vi "RT Loop - System Health and FPGA Monitoring.vi"(10 "FPGA VI Reference Out 2":refnum<k20>, 11 "Message Queue":refnum<queue>) -> (3 "x*y":dbl)   [LabVIEW 2017]
doc: "Send RT diagnostic information and FPGA monitoring data to UI Main VI."
uses:
  UI Error Handlers/support/Message Queue/Message Cluster.ctl
  controls/CPU Loads.ctl
  controls/FPGA State.ctl
  Globals/Global - Configuration Options.vi
  Globals/Global - All RT Loop Stop.vi
  <vilib>/Utility/error.llb/Error Cluster From Error Code.vi
  <vilib>/rvi/errors/niLvFpgaAdjustHostInterfaceError.vi
  <vilib>/nisyscfg/Close (System).vi
  <vilib>/rvi/interface/nirviReadWriteControl/nirviReadWriteControl.xnode
  <vilib>/NI_Real-Time Target Support.lvlib
  <vilib>/nisyscfg/nisyscfg.lvlib
  <resource>/objmgr/nisysapi.rc
  NiFpgaLv.dll
  <vilib>/rvi/interface/Simulation/niFpgaSimulationCallBeginRW.vi
  UI Error Handlers/support/Message Queue/Message Queue.lvlib
panel:
  out "x = y?":bool
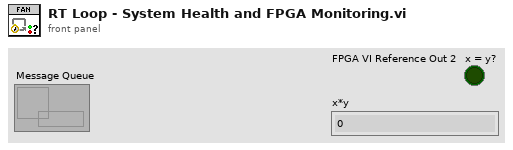
[diagram p1: front panel]
types:
  T1 = typedef "NI_Real-Time Target Support.lvlib/RT CPU Load.ctl" = cluster{"Total (%)":dbl, "Time Critical (%)":dbl, "Timed Structures (%)":dbl, "High (%)":dbl, "Above Normal (%)":dbl, "Normal (%)":dbl, "Background (%)":dbl, "Idle (%)":dbl, "ISR (%)":dbl}
  T2 = cluster{"Tool data":cluster{"Number of teeth":sgl}, "Cutting data":cluster{"rpm":sgl}, "Limits":cluster{"Magnitude threshold":sgl, "Tolerance":sgl}, "G1 status":cluster{"G1 trigger":bool}}
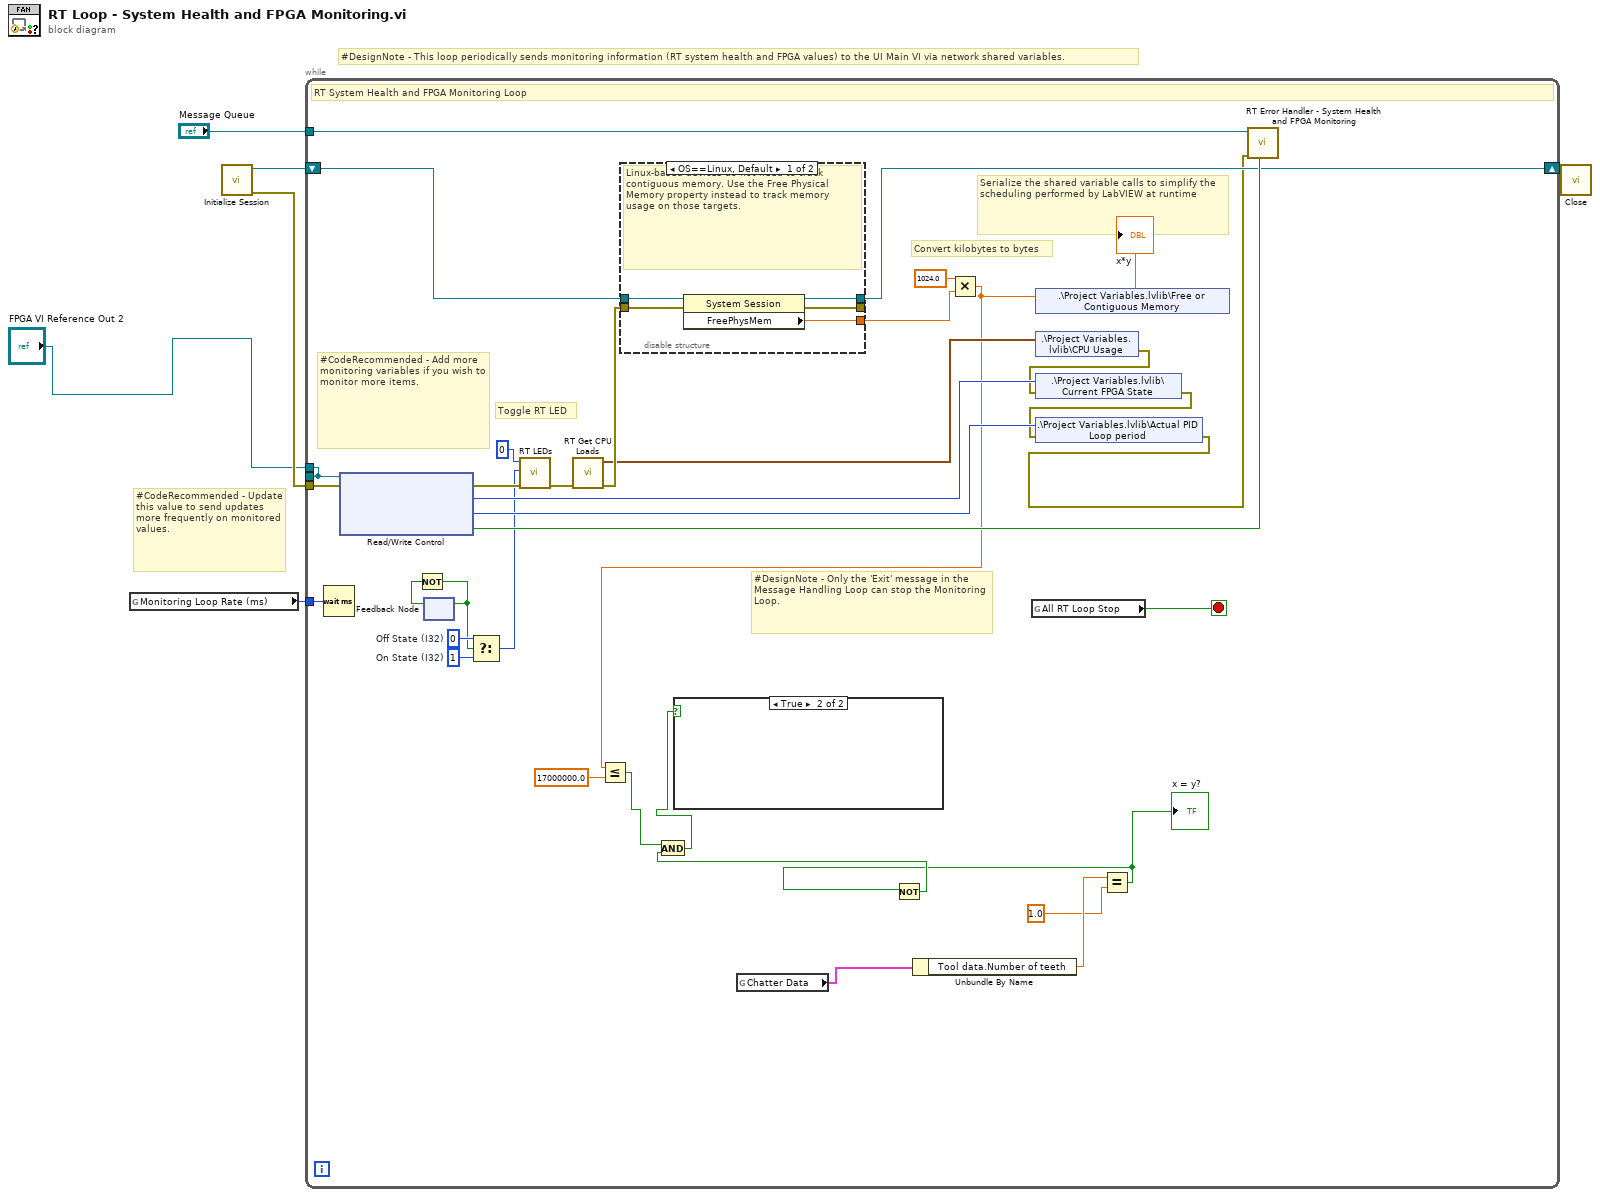
[diagram p0: block diagram]
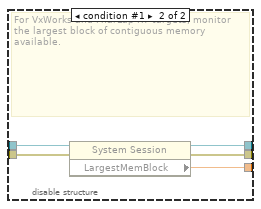
[diagram p3: hidden frame]
diagram:
  # "#CodeRecommended - Update this value to send updates more frequently on monitored values."
  # "#DesignNote - This loop periodically sends monitoring information (RT system health and FPGA values) to the UI Main VI via network shared variables."
  n1 = global read "Global - Configuration Options.vi" "Monitoring Loop Rate (ms)"() -> (w5:u32)
  n2 = call <vilib>:"Initialize Session.vi"() -> ("error out"=w2:errorcluster, "Session out"=w4:refnum<k21>)  [unwired: 10 in]
  n3 = while {
    tunnel: "Message Queue" -> [w37]
    tunnel: [w17] -> _
    tunnel: w5 -> [w36]
    shift-right: [w25] -> w3
    shift-left: w4 -> [w28]
    tunnel: w2 -> [w32]
    tunnel: "FPGA VI Reference Out 2" -> [w17]
    stop <- w38 stop-if-true
    w21 = 1  # On State (I32)
    w22 = 0  # Off State (I32)
    # "Convert kilobytes to bytes"
    # "Toggle RT LED"
    # "Serialize the shared variable calls to simplify the scheduling performed by LabVIEW at runtime"
    # "#CodeRecommended - Add more monitoring variables if you wish to monitor more items."
    # "#DesignNote - Only the 'Exit' message in the  Message Handling Loop can stop the Monitoring Loop."
    # "RT System Health and FPGA Monitoring Loop"
    n4 = Wait (ms)(milliseconds to wait=w36) -> ()  [unwired: 1 out]
    n5 = xnode "Read/Write Control"("FPGA VI Reference In"=w17, "error in"=w32) -> ("error out"=w30:errorcluster, "Current FPGA State"=w39:enum16{"Safe State", "Control (PID)"}, "PID Loop Period (tick)"=w40:u32, "Input Error"=w35:bool)  [unwired: 1 out]
    n6 = feedback #1() -> (w19:bool)  [unwired: 1 in]
    n7 = Not(x=w19) -> (.not. x?=w20:bool)
    n8 = feedback-in #1(w20) -> ()
    n9 = Select(t=w22, s=w20, f=w21) -> (s? t:f=w18:i32)
    n10 = call <vilib>:"RT LEDs.vi"("error in (no error)"=w30, "State"=w18, "LED Num"=0) -> ("error out"=w29:errorcluster)  [unwired: 3 in, 1 out]
    n11 = call <vilib>:"RT Get CPU Loads.vi"("error in (no error)"=w29) -> ("error out"=w26:errorcluster, "CPU loads"=w23:T1[])  [unwired: 9 in]
    n12 = disable-structure shown="OS==Linux, Default" {
      disable-tunnel: w28 -> [w45 w50]
      disable-tunnel: w26 -> [w44 w49]
      disable-tunnel: [w43 w48] -> w25
      disable-tunnel: [w42 w47] -> _
      disable-tunnel: [w41 w46] -> w24
      frame condition #0 (active) {
        # "Linux-based devices do not need to track contiguous memory. Use the Free Physical Memory property instead to track memory usage on those targets."
        n13 = property class="System Session"(reference=w45, error in=w44) -> (reference out=w43:refnum<k21>, error out=w42:errorcluster, "FreePhysMem"=w41:dbl)
      }
      frame condition #1 {
        # "For VxWorks and PharLap RT targets, monitor the largest block of contiguous memory available."
        n14 = property class="System Session"(reference=w50, error in=w49) -> (reference out=w48:refnum<k21>, error out=w47:errorcluster, "LargestMemBlock"=w46:dbl)
      }
    }
    n15 = global read "Global - Configuration Options.vi" "Chatter Data"() -> (w10:T2)
    n16 = Unbundle By Name(w10) -> ("Tool data.Number of teeth"=w9:sgl)
    n17 = Multiply(x=1024.0, y=w24) -> (x*y=w15:dbl)
    "x*y" <- w15
    n18 = Less Or Equal?(x=w15, y=17000000.0) -> (x <= y?=w13:bool)
    n19 = global read "Global - All RT Loop Stop.vi" "All RT Loop Stop"() -> (w38:bool)
    n20 = shared-variable ".\\Project Variables.lvlib\\Free or Contiguous Memory"(w15) -> ()  [unwired: 1 in, 1 out]
    n21 = shared-variable ".\\Project Variables.lvlib\\CPU Usage"(w23) -> (error out=w33:errorcluster)  [unwired: 1 in]
    n22 = shared-variable ".\\Project Variables.lvlib\\Current FPGA State"(w39, error in=w33) -> (error out=w34:errorcluster)
    n23 = shared-variable ".\\Project Variables.lvlib\\Actual PID Loop period"(w40, error in=w34) -> (error out=w16:errorcluster)
    n24 = Equal?(x=w9, y=1.0) -> (x = y?=w7:bool)
    "x = y?" <- w7
    n25 = Not(x=w7) -> (.not. x?=w12:bool)
    n26 = And(x=w13, y=w12) -> (x .and. y?=w11:bool)
    n27 = case shown="True" w11 {
      frame False {
      }
      frame True {
      }
    }
    n28 = call "RT Error Handler - System Health and FPGA Monitoring.vi"("Input Error (FPGA)"=w35, "error in (no error)"=w16, "Message Queue"=w37) -> ()  [unwired: 8 in, 1 out]
  }
  n29 = call-poly <vilib>:"Close.vi"("Session in"=w3) -> ()  [unwired: 10 in, 1 out]
